vi "Assert Array Count.vi"(4 "Execution time (s)":dbl=-1.0, 5 "Assert Only? (F)":bool, 6 "error code (1)":i32=1, 7 "Label (\"\")":string, 8 "error in (no error)":errorcluster, 9 "Register with caller test (F)":bool, 10 "Count":i32, 11 "Array":variant) -> (0 "error out":errorcluster, 2 "Properties.Assert":refnum<class "Properties.Assert.lvclass">)   [LabVIEW 2013, in "Caraya.lvlib" / "Assert.lvclass"]
doc: "Asserts that an array contains a specific number of elements."
uses:
  Assert.lvclass
  Properties.Assert/Properties.Assert.lvclass
  Properties/Properties.lvclass
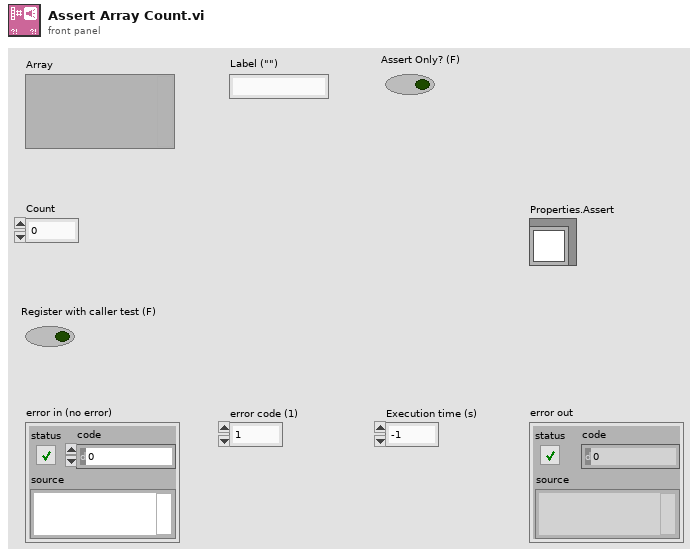
[diagram p1: front panel]
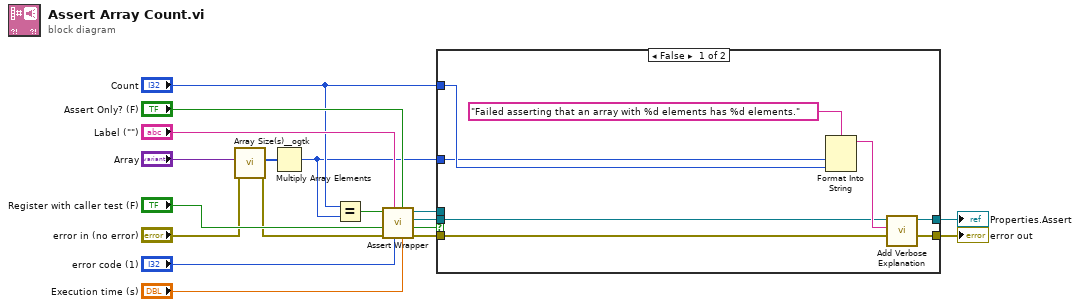
[diagram p0: block diagram]
diagram:
  n1 = call <userlib>:"Array Size(s)__ogtk.vi"("error in (no error)"="error in (no error)", "Array"="Array") -> ("error out"=w4:errorcluster, "Size(s)"=w3:u32[])  [unwired: 7 in, 1 out]
  n2 = Multiply Array Elements(1:w3) -> (0:w1:u32)
  n3 = Equal?(x="Count", y=w1) -> (x = y?=w7:bool)
  n4 = call "Assert Wrapper.vi"("Execution time (s)"="Execution time (s)", "Assert Only? (F)"="Assert Only? (F)", "error code (1)"="error code (1)", "Label"="Label (\"\")", "error in (no error)"=w4, "Register with caller test (F)"="Register with caller test (F)", "Assert?"=w7) -> ("error out"=w9:errorcluster, "Verbose"=w13:bool, "Properties.Assert"=w11:refnum<class "Properties.Assert.lvclass">, "Assert out"=w12:refnum<class "Assert.lvclass">)  [unwired: 1 in]
  n5 = case shown="False" w13 {
    tunnel: w12 -> [_ _]
    tunnel: w11 -> [w22 w28]
    tunnel: [w24 w27] -> w10
    tunnel: w9 -> [w25 w27]
    tunnel: "Count" -> [w26 _]
    tunnel: [w21 w28] -> w8
    tunnel: w1 -> [w19 _]
    frame False {
      n6 = Format Into String(format string="Failed asserting that an array with %d elements has %d elements.", w19, w26) -> (resulting string=w23:string)  [unwired: 2 in, 1 out]
      n7 = call "Add Verbose Explanation.vi"("error in (no error)"=w25, "Verbose Explanation"=w23, "Properties"=w22) -> ("error out"=w24:errorcluster, "Properties"=w21:refnum<class "Properties.Assert.lvclass">)  [unwired: 7 in]
    }
    frame True {
    }
  }
  "error out" <- w10
  "Properties.Assert" <- w8
